vi "Decimate Fcurve.vi"(0 "Fcurve":T1, 1 "decimating factor":i32=1, 5 "error in (no error)":errorcluster) -> (14 "Decimated Fcurve":cluster{"X":dbl[], "Y":dbl[]}[](array[cluster]), 19 "error out":errorcluster)   [LabVIEW 2019, in "Force Curve_tdms.lvclass"]
uses:
  Force Curve_tdms.lvclass
  Force Curve data.ctl
  <vilib>/Analysis/2dsp.llb/Decimate (continuous, DBL).vi
  <vilib>/Analysis/NI_AALPro.lvlib
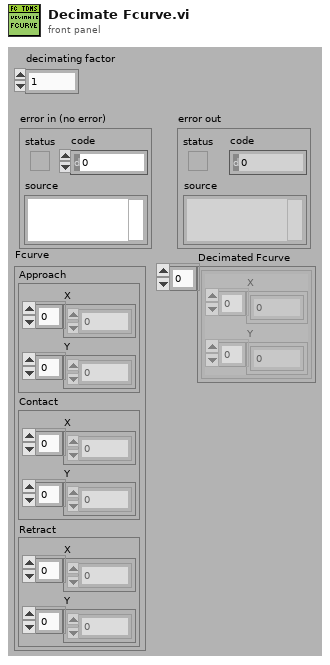
[diagram p1: front panel]
types:
  T1 = typedef "Force Curve_tdms.lvclass/Force Curve data.ctl" = cluster{"Approach":cluster{"X":dbl[], "Y":dbl[]}, "Contact":cluster{"X":dbl[], "Y":dbl[]}, "Retract":cluster{"X":dbl[], "Y":dbl[]}}
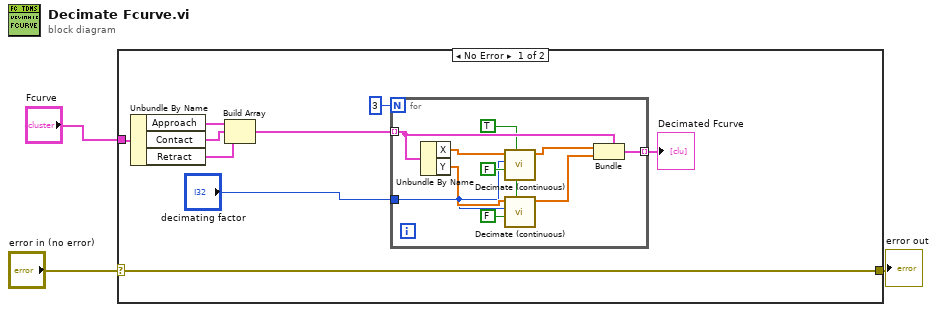
[diagram p0: block diagram]
diagram:
  n1 = case shown="No Error" "error in (no error)" {
    selector: "error in (no error)" -> [w12 w23]
    tunnel: [w12 w23] -> w2
    tunnel: "Fcurve" -> [w5 _]
    frame No Error {
      n2 = Unbundle By Name(w5) -> ("Approach"=w10:cluster{"X":dbl[], "Y":dbl[]}, "Contact"=w9:cluster{"X":dbl[], "Y":dbl[]}, "Retract"=w8:cluster{"X":dbl[], "Y":dbl[]})
      n3 = Build Array(w10, w9, w8) -> (w7:cluster{"X":dbl[], "Y":dbl[]}[])
      n4 = for {
        N: 3 -> [_]
        tunnel: w7 -> [w21] mode=indexing
        tunnel: "decimating factor" -> [w13]
        tunnel: [w22] -> w4 mode=indexing
        w16 = TRUE ("reset")
        n5 = Unbundle By Name(w21) -> ("X"=w20:dbl[], "Y"=w18:dbl[])
        n6 = call-poly <vilib>:"Decimate (continuous).vi"("reset"=w16, "averaging"=FALSE, "decimating factor"=w13, "X"=w20) -> ("Decimated Array"=w19:dbl[])  [unwired: 6 in, 1 out]
        n7 = call-poly <vilib>:"Decimate (continuous).vi"("reset"=w16, "averaging"=FALSE, "decimating factor"=w13, "X"=w18) -> ("Decimated Array"=w17:dbl[])  [unwired: 6 in, 1 out]
        n8 = Bundle(cluster=w21, "X"=w19, "Y"=w17) -> (w22:cluster{"X":dbl[], "Y":dbl[]})
      }
      "Decimated Fcurve" <- w4
    }
    frame Error {
    }
  }
  "error out" <- w2
